vi "End.vi"(8 "error in (no error)":errorcluster, 11 "Channel in":refnum<class "SPARC4_Channel.lvclass">) -> (0 "error out":errorcluster, 3 "Channel out":refnum<class "SPARC4_Channel.lvclass">)   [LabVIEW 2018, in "SPARC4_Channel.lvclass"]
doc: "End the ACS execution \n\nThis function is responsible for eding the ACS execution correctly"
uses:
  SPARC4_Channel.lvclass
  SPARC4_Channel.lvclass/SPARC4_Channel.ctl
  Sim_Ixon_Ultra/Sim_Ixon_Ultra.lvclass
  C:/Users/Denis/Desktop/S4ACS/S4ACS/Sim_CCD/Sim_CCD.lvclass
  Sim_CCD/Sim_CCD.lvclass
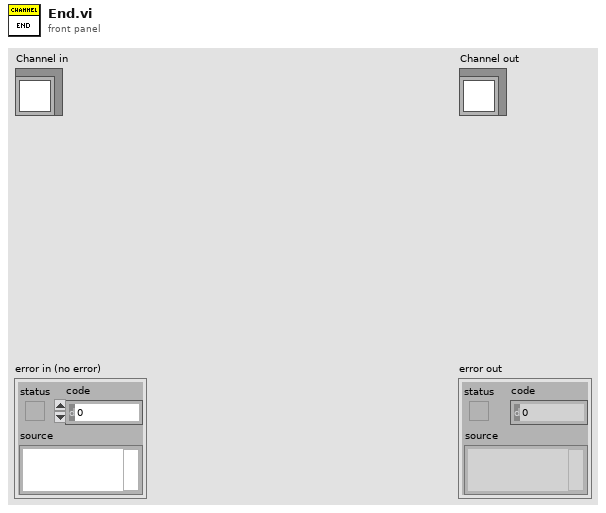
[diagram p1: front panel]
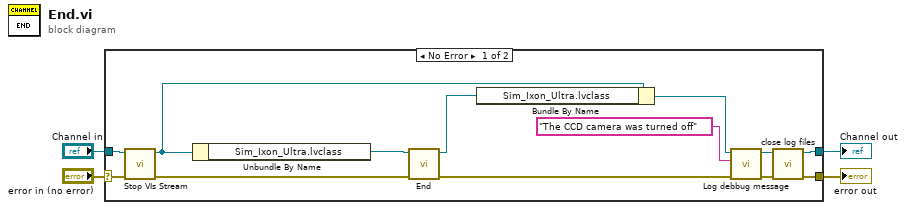
[diagram p0: block diagram]
diagram:
  n1 = case shown="No Error" "error in (no error)" {
    selector: "error in (no error)" -> [w5 w19]
    tunnel: [w12 w19] -> w3
    tunnel: [w13 w18] -> w1
    tunnel: "Channel in" -> [w6 w18]
    frame No Error {
      n2 = call "Stop VIs Stream.vi"("error in (no error)"=w5, "Channel in"=w6) -> ("error out"=w14:errorcluster, "Channel out"=w15:refnum<class "SPARC4_Channel.lvclass">)  [unwired: 8 in]
      n3 = Unbundle By Name(w15) -> ("Sim_Ixon_Ultra.lvclass"=w17:refnum<class "Sim_Ixon_Ultra.lvclass">)
      n4 = call "End.vi"("error in (no error)"=w14, "Simulated_CCD_Camera in"=w17) -> ("error out"=w8:errorcluster, "Simulated_CCD_Camera out"=w16:refnum<class "Sim_Ixon_Ultra.lvclass">)  [unwired: 8 in]
      n5 = Bundle By Name(cluster=w15, "Sim_Ixon_Ultra.lvclass"=w16) -> (w11:refnum<class "SPARC4_Channel.lvclass">)
      n6 = call "Log debbug message.vi"("error in (no error)"=w8, "String"="The CCD camera was turned off", "Channel in"=w11) -> ("error out"=w9:errorcluster, "Channel out"=w10:refnum<class "SPARC4_Channel.lvclass">)  [unwired: 7 in]
      n7 = call "close log files.vi"("error in (no error)"=w9, "Channel in"=w10) -> ("error out"=w12:errorcluster, "Channel out"=w13:refnum<class "SPARC4_Channel.lvclass">)  [unwired: 8 in]
    }
    frame Error {
    }
  }
  "error out" <- w3
  "Channel out" <- w1
